vi "InitImageDisplay.vi"(8 "error in (no error)":errorcluster, 10 "payload data type":T1(ring), 11 "SI channel":string) -> (0 "error out":errorcluster, 2 "Image Out Color":T2, 3 "Image Out Grayscale":T2)   [LabVIEW 2025]
uses:
  <vilib>/vision/Image Controls.llb/IMAQ Image.ctl
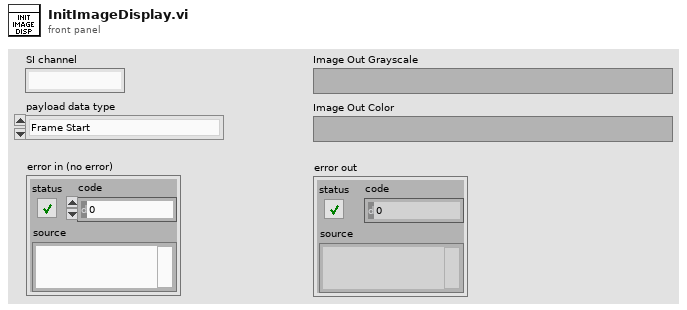
[diagram p1: front panel]
types:
  T1 = enum8{"Frame Start", "Frame End", "Line Start", "Line End", "End of Transmission", "Reserved 0", "Reserved 1", "Reserved 2", "Generic Short Packet 1", "Generic Short Packet 2", "Generic Short Packet 3", "Generic Short Packet 4", "Generic Short Packet 5", "Generic Short Packet 6", "Generic Short Packet 7", "Generic Short Packet 8", "Null", "Blanking Data", "Embedded 8-bit non Image Data", "Generic Long Packet 1", "Generic Long Packet 2", "Generic Long Packet 3", "Generic Long Packet 4", "Reserved 3", "YUV420 8-bit", "YUV420 10-bit", "Legacy YUV420 8-bit", "Reserved 4", "YUV420 8-bit Chroma Shifted", "YUV420 10-bit Chroma Shifted", "YUV422 8-bit", "YUV422 10-bit", "RGB444", "RGB555", "RGB565", "RGB666", "RGB888", "Reserved 5", "Reserved 6", "RAW 24", "RAW 6", "RAW 7", "RAW 8", "RAW 10", "RAW 12", "RAW 14", "RAW 16", "RAW 20", "User Defined 8-bit Data 1", "User Defined 8-bit Data 2", "User Defined 8-bit Data 3", "User Defined 8-bit Data 4", "User Defined 8-bit Data 5", "User Defined 8-bit Data 6", "User Defined 8-bit Data 7", "User Defined 8-bit Data 8", "USL Command", "Reserved 7", "Reserved 8", "Reserved 9", "Reserved 10", "Reserved 11", "Reserved 12", "LRTE EPD Spacer"}
  T2 = typedef "IMAQ Image.ctl" = refnum<image>
  T3 = typedef "Image Type" = u32
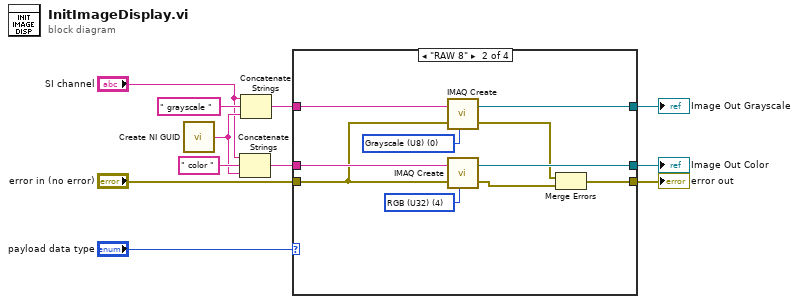
[diagram p0: block diagram]
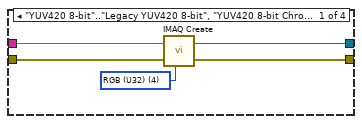
[diagram p2: hidden frame]
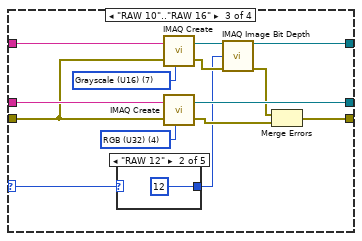
[diagram p3: hidden frame]
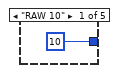
[diagram p4: hidden frame]
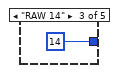
[diagram p5: hidden frame]
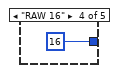
[diagram p6: hidden frame]
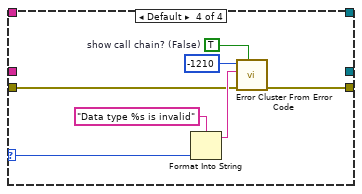
[diagram p8: hidden frame]
diagram:
  n1 = call <vilib>:"Create NI GUID.vi"() -> ("NI GUID"=w7:string)
  n2 = Concatenate Strings("SI channel", " color " ("Image Name"), w7) -> (w8:string)
  n3 = Concatenate Strings("SI channel", " grayscale " ("Image Name"), w7) -> (w10:string)
  n4 = case shown="\"RAW 8\"" "payload data type" {
    selector: "payload data type" -> [_ _ w34 w48]
    tunnel: w10 -> [_ w26 w40 _]
    tunnel: w8 -> [w15 w25 w39 _]
    tunnel: "error in (no error)" -> [w14 w24 w38 w46]
    tunnel: [w12 w23 w37 w45] -> w4
    tunnel: [w13 w22 w36 _] -> w2
    tunnel: [_ w21 w35 _] -> w3
    frame "YUV420 8-bit".."Legacy YUV420 8-bit", "YUV420 8-bit Chroma Shifted".."YUV422 10-bit", "RGB565".."RGB888" {
      w16 = T3 4 items=["Grayscale (U8)", "Grayscale (I16)", "Grayscale (SGL)", "Complex (CSG)", "RGB (U32)", "HSL (U32)", "RGB (U64)", "Grayscale (U16)"] ("Image Type")
      n5 = call "IMAQ Create"("Image Name"=w15, "Image Type"=w16, "error in (no error)"=w14) -> ("New Image"=w13:T2, "error out"=w12:errorcluster)  [unwired: 2 in]
    }
    frame "RAW 8" {
      w19 = T3 4 items=["Grayscale (U8)", "Grayscale (I16)", "Grayscale (SGL)", "Complex (CSG)", "RGB (U32)", "HSL (U32)", "RGB (U64)", "Grayscale (U16)"] ("Image Type")
      w20 = T3 0 items=["Grayscale (U8)", "Grayscale (I16)", "Grayscale (SGL)", "Complex (CSG)", "RGB (U32)", "HSL (U32)", "RGB (U64)", "Grayscale (U16)"] ("Image Type")
      n6 = call "IMAQ Create"("Image Name"=w26, "Image Type"=w20, "error in (no error)"=w24) -> ("New Image"=w21:T2, "error out"=w17:errorcluster)  [unwired: 2 in]
      n7 = call "IMAQ Create"("Image Name"=w25, "Image Type"=w19, "error in (no error)"=w24) -> ("New Image"=w22:T2, "error out"=w18:errorcluster)  [unwired: 2 in]
      n8 = Merge Errors(w17, w18) -> (w23:errorcluster)
    }
    frame "RAW 10".."RAW 16" {
      w32 = T3 4 items=["Grayscale (U8)", "Grayscale (I16)", "Grayscale (SGL)", "Complex (CSG)", "RGB (U32)", "HSL (U32)", "RGB (U64)", "Grayscale (U16)"] ("Image Type")
      w33 = T3 7 items=["Grayscale (U8)", "Grayscale (I16)", "Grayscale (SGL)", "Complex (CSG)", "RGB (U32)", "HSL (U32)", "RGB (U64)", "Grayscale (U16)"] ("Image Type")
      n9 = case shown="\"RAW 12\"" w34 {
        tunnel: [u32 10 ("Bit Depth (0)") u32 12 ("Bit Depth (0)") u32 14 ("Bit Depth (0)") u32 16 ("Bit Depth (0)") _] -> w27
        frame "RAW 10" {
        }
        frame "RAW 12" {
        }
        frame "RAW 14" {
        }
        frame "RAW 16" {
        }
        frame Default {
        }
      }
      n10 = call "IMAQ Create"("Image Name"=w40, "Image Type"=w33, "error in (no error)"=w38) -> ("New Image"=w30:T2, "error out"=w29:errorcluster)  [unwired: 2 in]
      n11 = call "IMAQ Create"("Image Name"=w39, "Image Type"=w32, "error in (no error)"=w38) -> ("New Image"=w36:T2, "error out"=w31:errorcluster)  [unwired: 2 in]
      n12 = call "IMAQ Image Bit Depth"("Image"=w30, "Bit Depth (0)"=w27, "error in (no error)"=w29) -> ("Image Out"=w35:T2, "error out"=w28:errorcluster)  [unwired: 10 in, 1 out]
      n13 = Merge Errors(w28, w31) -> (w37:errorcluster)
    }
    frame Default {
      w50 = TRUE  # show call chain? (False)
      n14 = Format Into String(format string="Data type %s is invalid" ("error message (\"\")"), w48) -> (resulting string=w47:string)  [unwired: 2 in, 1 out]
      n15 = call <vilib>:"Error Cluster From Error Code.vi"("show call chain? (False)"=w50, "error in (no error)"=w46, "error message (\"\")"=w47, "error code (0)"=-1210) -> ("error out"=w45:errorcluster)  [unwired: 5 in]
    }
  }
  "error out" <- w4
  "Image Out Grayscale" <- w3
  "Image Out Color" <- w2
